vi "FTW-Endpoint-Ask.vi"(0 "FTW Endpoint":refnum<class "FTW-Endpoint.lvclass">, 5 "Request Header":string, 7 "Request Body":string, 9 "Timeout":i32=1000 format="%dmsec", 11 "error in":errorcluster) -> (4 "FTW Endpoint out":refnum<class "FTW-Endpoint.lvclass">, 6 "Response Header":string, 8 "Response Body":string, 10 "Timed out?":bool, 13 "Response Message":T1, 14 "Roundtrip Time":dbl format="%.6fsec", 15 "error out":errorcluster)   [LabVIEW 2015, in "FTW-Endpoint.lvclass"]
uses:
  FTW-Endpoint.lvclass
  Payload/FTW-MessagePayload.ctl
panel:
  # "Inputs"
  # "Outputs"
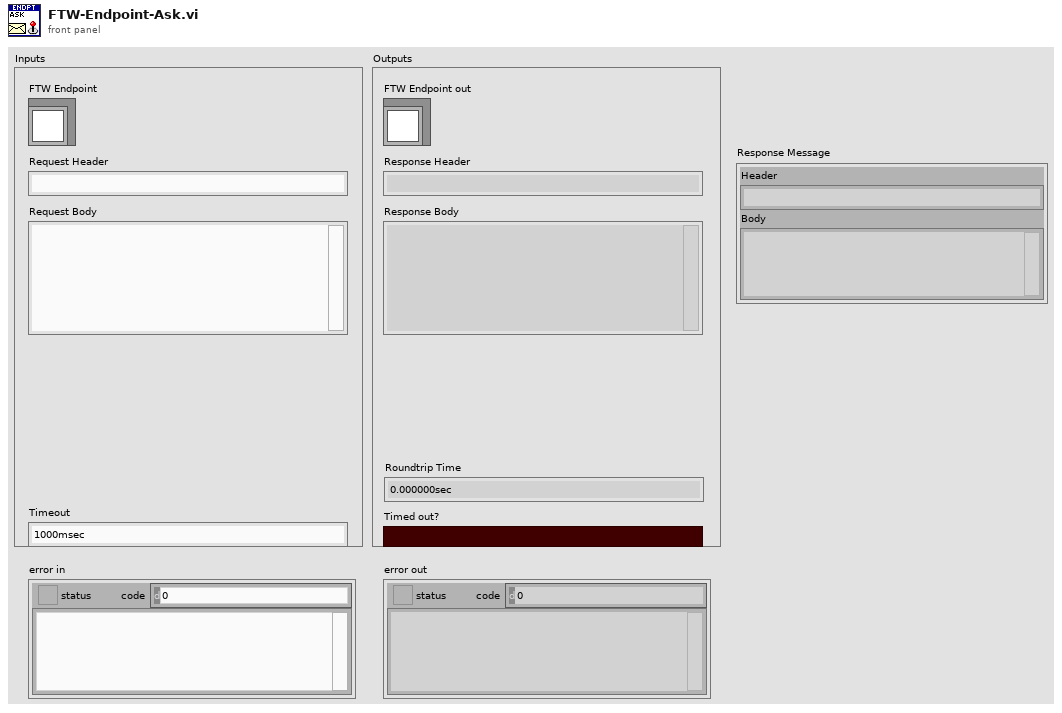
[diagram p1: front panel]
types:
  T1 = typedef "FTW-MessagePayload.ctl" = cluster{"Header":string, "Body":string, "FTW: Sender Identity":string, "FTW: Reply Address":string, "FTW: Reply Error":errorcluster}
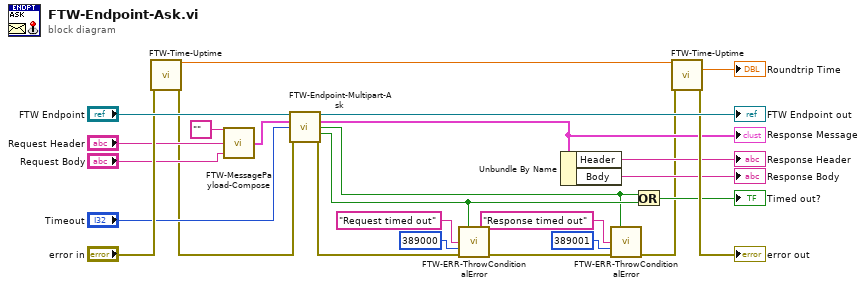
[diagram p0: block diagram]
diagram:
  n1 = call "FTW-Time-Uptime.vi"("error in"="error in") -> ("Current Uptime"=w16:dbl, "error out"=w18:errorcluster)  [unwired: 12 in, 1 out]
  n2 = call "FTW-MessagePayload-Compose.vi"("Message Body"="Request Body", "Message Header"="Request Header", "Sender Identity"="" ("empty string")) -> ("Message"=w14:T1)  [unwired: 1 in]
  n3 = call-dynamic "FTW-Endpoint-Multipart-Ask.vi"("FTW Endpoint"="FTW Endpoint", "Message"=w14, "Read Timeout"="Timeout", "error in"=w18) -> ("FTW Endpoint out"=→"FTW Endpoint out":refnum<class "FTW-Endpoint.lvclass">, "Reply"=w10:T1, "Read Timed out?"=w3:bool, "Write Timed out?"=w6:bool, "error out"=w25:errorcluster)  [unwired: 7 in]
  "Response Message" <- w10
  n4 = call "FTW-ERR-ThrowConditionalError.vi"("Error Message"="Request timed out", "Error Code"=389000, "error in"=w25, "Throw Error?"=w6) -> ("error out"=w1:errorcluster)  [unwired: 11 in]
  n5 = Unbundle By Name(w10) -> ("Header"=→"Response Header":string, "Body"=→"Response Body":string)
  n6 = call "FTW-ERR-ThrowConditionalError.vi"("Error Message"="Response timed out", "Error Code"=389001, "error in"=w1, "Throw Error?"=w3) -> ("error out"=w2:errorcluster)  [unwired: 11 in]
  n7 = Or(x=w3, y=w6) -> (x .or. y?=→"Timed out?":bool)
  n8 = call "FTW-Time-Uptime.vi"("Previous Uptime"=w16, "error in"=w2) -> ("Elapsed Time"=→"Roundtrip Time":dbl, "error out"=→"error out":errorcluster)  [unwired: 11 in, 1 out]
